vi "Agilent SNA Set Sweep Type.vi"(6 "Channel":i8=1 min=1 max=99 step=1, 7 "Agilent SNA & SWP":T1, 8 "error in (no error)":errorcluster, 10 "Sweep Type":T3, 11 "VISA Resource Names":T2) -> (0 "error out":errorcluster, 3 "dup VISA Resource Names":T2)   [LabVIEW 2011]
doc: "This VI for the HP8753B is used to set the meausurement format."
uses:
  TypeDefs/Agilent SNA Sweep Type.ctl
  TypeDefs/Agilent SNA VISA.ctl
  TypeDefs/Agilent SNA Instrument Info.ctl
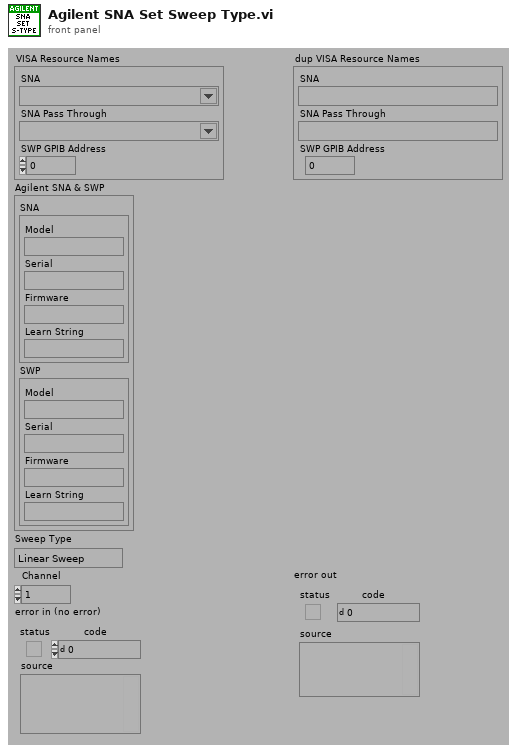
[diagram p1: front panel]
types:
  T1 = typedef "Agilent SNA Instrument Info.ctl" = cluster{"SNA":cluster{"Model":string, "Serial":string, "Firmware":string, "Learn String":string}, "SWP":cluster{"Model":string, "Serial":string, "Firmware":string, "Learn String":string}}
  T2 = typedef "Agilent SNA VISA.ctl" = cluster{"SNA":refnum<visa-resource-name>, "SNA Pass Through":refnum<visa-resource-name>, "SWP GPIB Address":i32}
  T3 = typedef "Agilent SNA Sweep Type.ctl" = enum32{"Linear Sweep", "CW Time Sweep", "Frequency List"}
  T4 = typedef "Agilent SNA Model.ctl" = enum16{"Not Supported", "8757X"}
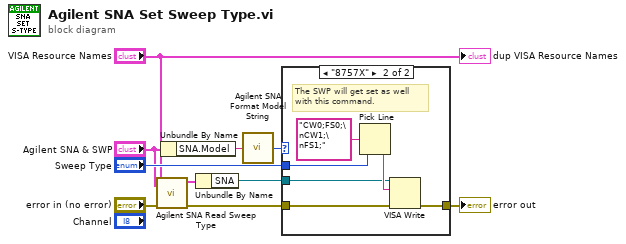
[diagram p0: block diagram]
diagram:
  n1 = call "Agilent SNA Read Sweep Type.vi"("Agilent SNA & SWP"="Agilent SNA & SWP", "error in (no error)"="error in (no error)", "VISA Resource Names"="VISA Resource Names") -> ("error out"=w8:errorcluster, "dup VISA Resource Names"=w3:T2)  [unwired: 1 in, 6 out]
  n2 = Unbundle By Name("Agilent SNA & SWP") -> ("SNA.Model"=w6:string)
  n3 = Unbundle By Name(w3) -> ("SNA"=w2:refnum<visa-resource-name>)
  n4 = call "Agilent SNA Format Model String.vi"("Model String"=w6) -> ("Model"=w4:T4)
  n5 = case shown="\"8757X\"" w4 {
    tunnel: [w11 w17] -> w10
    tunnel: w8 -> [w11 w15]
    tunnel: "Sweep Type" -> [_ w14]
    tunnel: w2 -> [_ w12]
    frame "Not Supported", Default {
    }
    frame "8757X" {
      # "The SWP will get set as well\nwith this command."
      n6 = Pick Line(multi-line string="CW0;FS0;\nCW1;\nFS1;", line index=w14) -> (output string=w16:string)  [unwired: 1 out]
      n7 = VISA Write(VISA resource name=w12, write buffer=w16, error in (no error)=w15) -> (error out=w17:errorcluster)  [unwired: 2 out]
    }
  }
  "error out" <- w10
  "dup VISA Resource Names" <- "VISA Resource Names"
